vi "DrawInvaders_Intensity.vi"(4 "Step_V":i32, 6 "Step_H":i32, 7 "Clear":bool, 9 "InitCluster_IN":T1, 11 "InvaderArray":bool[][](array[boolean])=[[TRUE, TRUE, TRUE, TRUE, TRUE, TRUE, TRUE, TRUE, TRUE, TRUE], [TRUE, TRUE, TRUE, TRUE, TRUE, TRUE, TRUE, TRUE, TRUE, TRUE], [TRUE, TRUE, TRUE, TRUE, TRUE, TRUE, TRUE, TRUE, TRUE, TRUE], [TRUE, TRUE, TRUE, TRUE, TRUE, TRUE, TRUE, TRUE, TRUE, TRUE], [TRUE, TRUE, TRUE, TRUE, TRUE, TRUE, TRUE, TRUE, TRUE, TRUE]]) -> (1 "InitCluster_OUT":T1, 3 "InvaderPosArray":T9(array[cluster]))   [LabVIEW 2022 SP3]
uses:
  InitCluster.ctl
  CharacterCluster.ctl
  <vilib>/picture/picture.llb/imagedata.ctl
  ShotInitCluster.ctl
  <vilib>/Utility/miscctls.llb/LVPositionTypeDef.ctl
  <vilib>/Utility/miscctls.llb/LVBoundsTypeDef.ctl
  ShotCluster.ctl
  move_dir_ud.ctl
panel:
  out "IG":u8[][](graph)
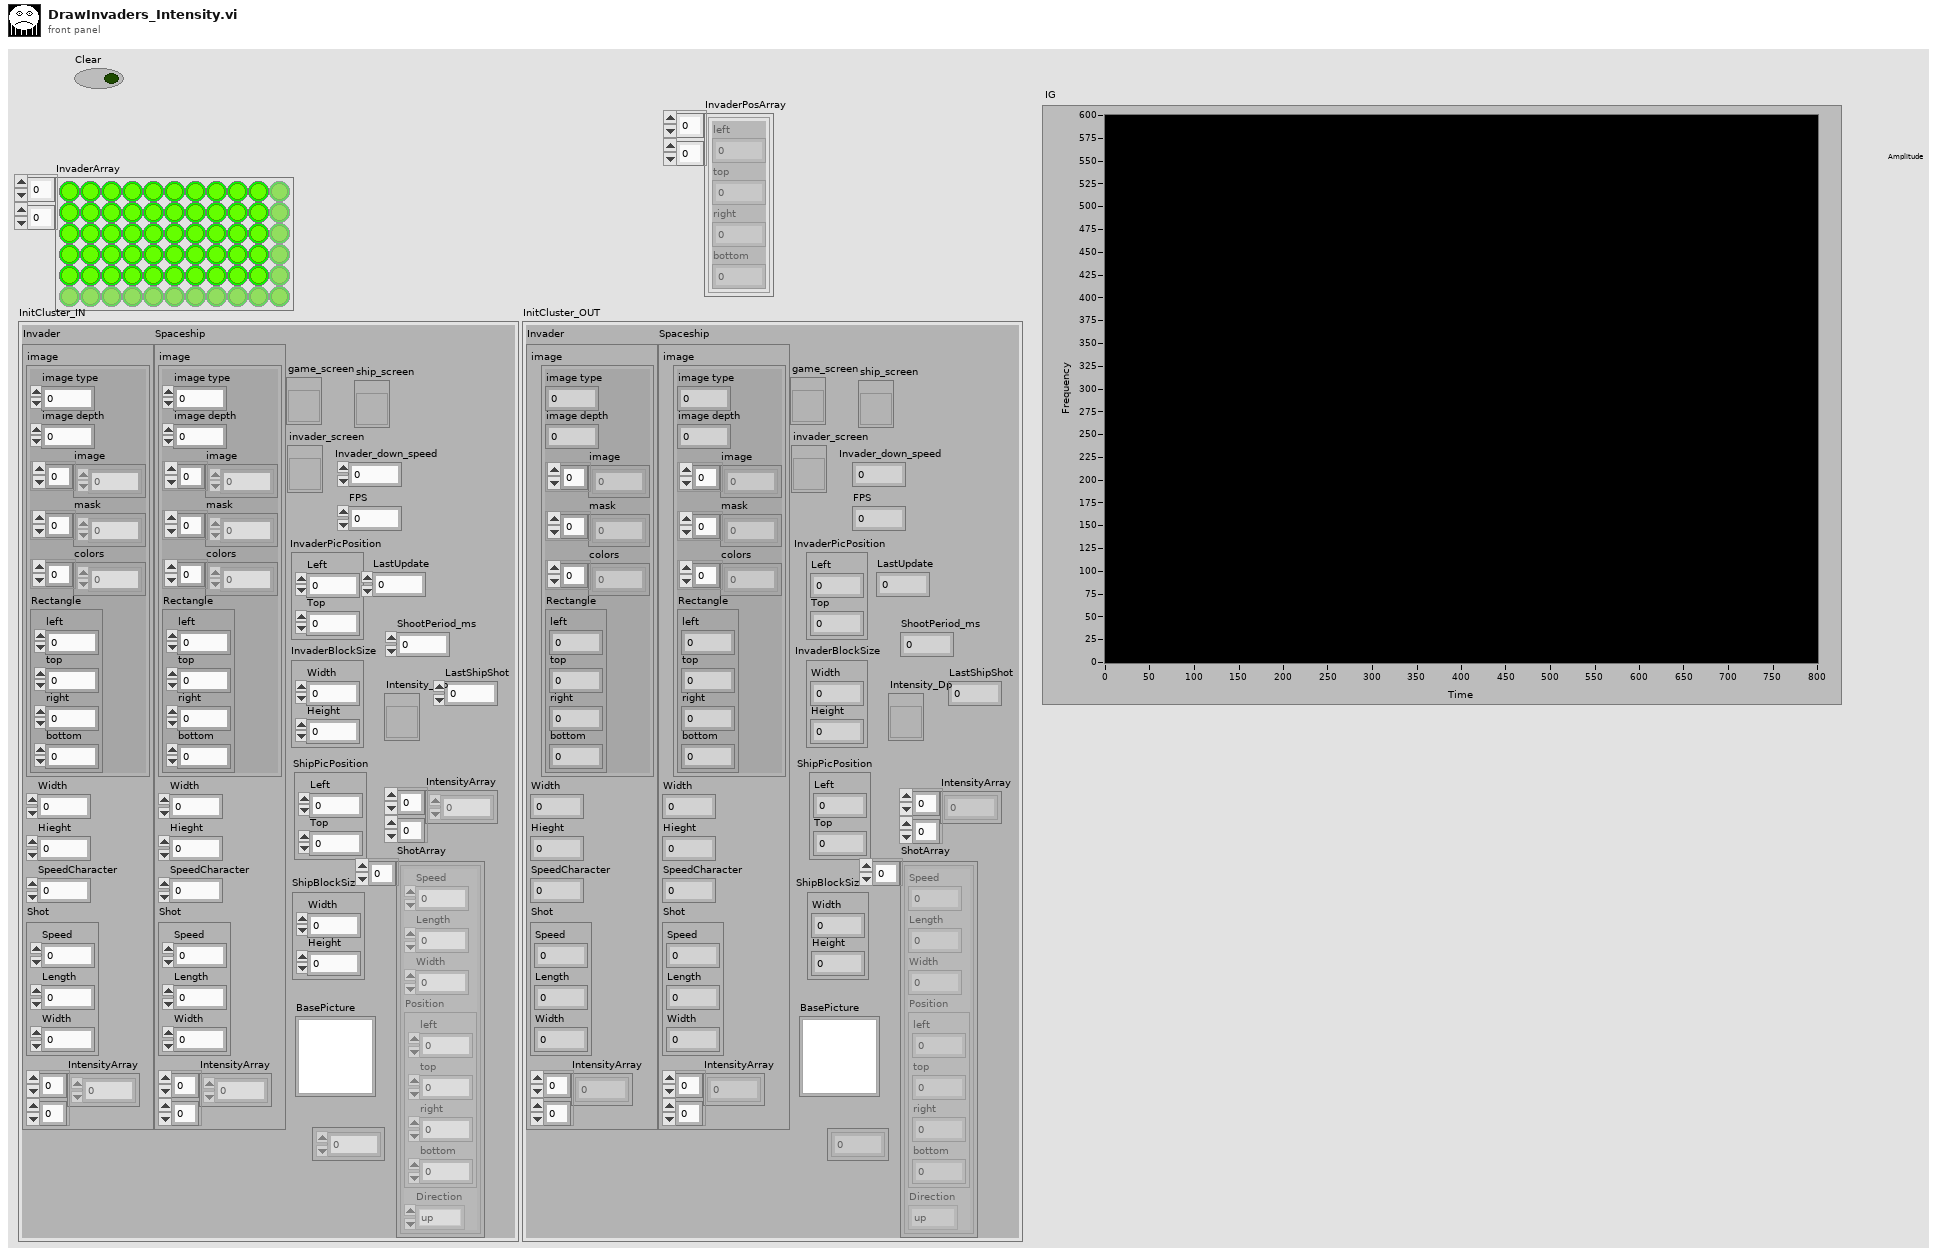
[diagram p1: front panel]
types:
  T1 = typedef "InitCluster.ctl" = cluster{"Invader":T2, "Spaceship":T2, "game_screen":refnum<vi>, "BasePicture":picture, "invader_screen":refnum<vi>, "InvaderPicPosition":T5, "Invader_down_speed":i16, "FPS":u16, "InvaderBlockSize":T6, "ship_screen":refnum<vi>, "ShipBlockSize":T6, "ShipPicPosition":T5, "LastUpdate":u32, "Intensity_Dp":refnum<vi>, "IntensityArray":u8[][], "ShotArray":T7[], "InvaderShotTimeArray":u32[], "ShootPeriod_ms":i32, "LastShipShot":u32}
  T2 = typedef "CharacterCluster.ctl" = cluster{"image":T3, "Width":u32, "Hieght":u32, "SpeedCharacter":u32, "Shot":T4, "IntensityArray":u8[][]}
  T3 = typedef "imagedata.ctl" = cluster{"image type":i32, "image depth":i32, "image":u8[], "mask":u8[], "colors":u32[], "Rectangle":cluster{"left":i16, "top":i16, "right":i16, "bottom":i16}}
  T4 = typedef "ShotInitCluster.ctl" = cluster{"Speed":u32, "Length":u32, "Width":u32}
  T5 = typedef "LVPositionTypeDef.ctl" = cluster{"Left":i32, "Top":i32}
  T6 = typedef "LVBoundsTypeDef.ctl" = cluster{"Width":u32, "Height":u32}
  T7 = typedef "ShotCluster.ctl" = cluster{"Speed":u32, "Length":u32, "Width":u32, "Position":cluster{"left":i16, "top":i16, "right":i16, "bottom":i16}, "Direction":T8}
  T8 = typedef "move_dir_ud.ctl" = enum16{"up", "down"}
  T9 = cluster{"left":i16, "top":i16, "right":i16, "bottom":i16}[][]
  T10 = cluster{"left":i16, "top":i16, "right":i16, "bottom":i16}
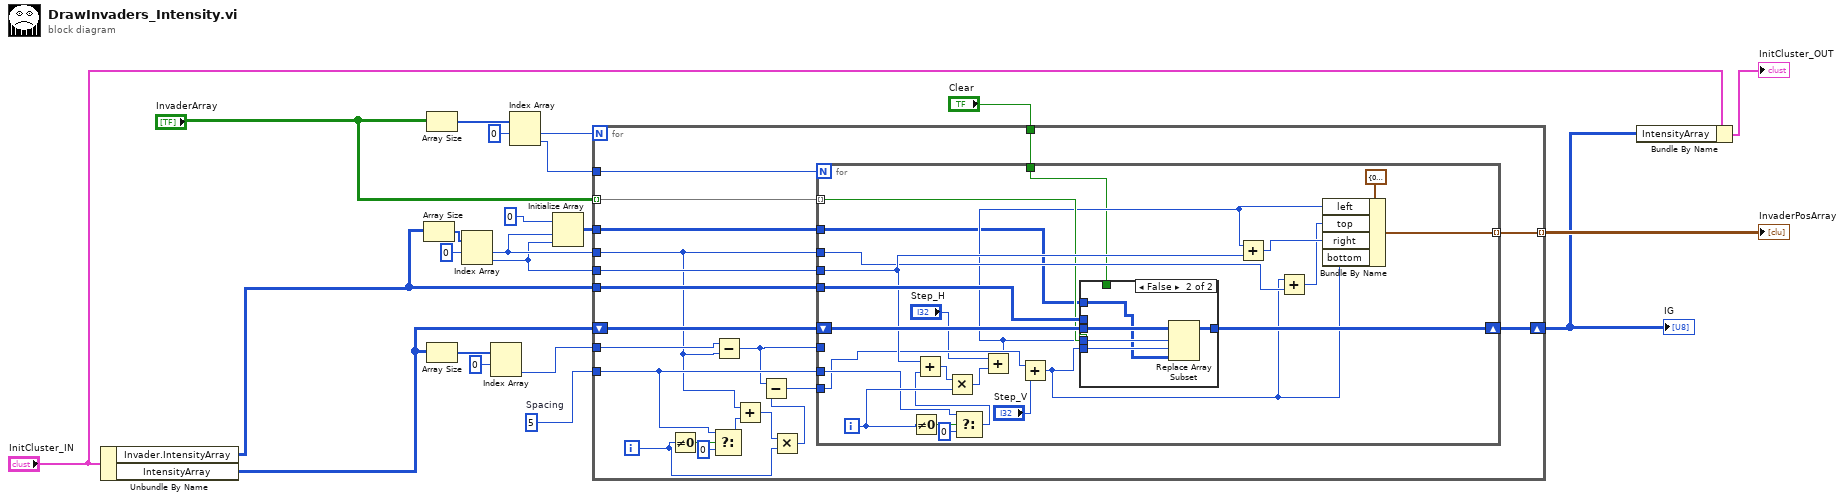
[diagram p0: block diagram]
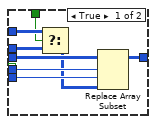
[diagram p2: hidden frame]
diagram:
  w22 = u8 5  # Spacing
  n1 = Unbundle By Name("InitCluster_IN") -> ("Invader.IntensityArray"=w12:u8[][], "IntensityArray"=w4:u8[][])
  n2 = Array Size(array=w12) -> (size(s)=w20:i32[])
  n3 = Array Size(array="InvaderArray") -> (size(s)=w18:i32[])
  n4 = Array Size(array=w4) -> (size(s)=w6:i32[])
  n5 = Index Array(array=w20, index #1=0 ("index")) -> (element #1=w11:i32, element #2=w10:i32)  [unwired: 1 in]
  n6 = Index Array(array=w6, index #1=0 ("index")) -> (element #2=w13:i32)  [unwired: 1 in, 1 out]
  n7 = Index Array(array=w18, index #1=0 ("index")) -> (element #1=w16:i32, element #2=w15:i32)  [unwired: 1 in]
  n8 = Initialize Array(u8 0, w11, w10) -> (w8:u8[][])
  n9 = for {
    N: w16 -> [_]
    tunnel: w12 -> [w42]
    shift-right: [w40] -> w1
    shift-left: w4 -> [w41]
    tunnel: w22 -> [w35]
    tunnel: w11 -> [w28]
    tunnel: w10 -> [w39]
    tunnel: w13 -> [w30]
    tunnel: [w27] -> w19 mode=indexing
    tunnel: w15 -> [w26]
    tunnel: "InvaderArray" -> [w25] mode=indexing
    tunnel: w8 -> [w24]
    tunnel: "Clear" -> [w23]
    i -> [w32]
    n10 = Not Equal To 0?(x=w32) -> (x != 0?=w37:bool)
    n11 = Select(t=w35, s=w37, f=u8 0) -> (s? t:f=w36:u8)
    n12 = Subtract(x=w30, y=w28) -> (x-y=w29:i32)
    n13 = Add(x=w28, y=w36) -> (x+y=w33:i32)
    n14 = Multiply(x=w33, y=w32) -> (x*y=w31:i32)
    n15 = Subtract(x=w29, y=w31) -> (x-y=w34:i32)
    n16 = for {
      N: w26 -> [_]
      tunnel: w42 -> [w64]
      tunnel: w35 -> [w60]
      shift-right: [w65] -> w40
      shift-left: w41 -> [w66]
      tunnel: w28 -> [w54]
      tunnel: w39 -> [w56]
      tunnel: w29 -> [_]
      tunnel: w34 -> [w50]
      tunnel: [w53] -> w27 mode=indexing
      tunnel: w25 -> [w51] mode=indexing
      tunnel: w24 -> [w44]
      tunnel: w23 -> [w43]
      i -> [w62]
      n17 = Not Equal To 0?(x=w62) -> (x != 0?=w61:bool)
      n18 = Select(t=w60, s=w61, f=u8 0) -> (s? t:f=w58:u8)
      n19 = Add(x=w56, y=w58) -> (x+y=w63:i32)
      n20 = Multiply(x=w63, y=w62) -> (x*y=w47:i32)
      n21 = Add(x="Step_H", y=w47) -> (x+y=w45:i32)
      n22 = Add(x=w50, y="Step_V") -> (x+y=w48:i32)
      n23 = case shown="False" w51 {
        tunnel: w66 -> [w74 w79]
        tunnel: [w73 w78] -> w65
        tunnel: w64 -> [w69 _]
        tunnel: w45 -> [w72 w77]
        tunnel: w48 -> [w71 w76]
        tunnel: w44 -> [w70 w75]
        tunnel: w43 -> [w68 _]
        frame True {
          n24 = Select(t=w70, s=w68, f=w69) -> (s? t:f=w67:u8[][])
          n25 = Replace Array Subset(array=w74, new element=w67, index (row)=w72, index (col)=w71) -> (w73:u8[][])
        }
        frame False {
          n26 = Replace Array Subset(array=w79, new element=w75, index (row)=w77, index (col)=w76) -> (w78:u8[][])
        }
      }
      n27 = Add(x=w45, y=w56) -> (x+y=w55:i32)
      n28 = Add(x=w48, y=w54) -> (x+y=w52:i32)
      n29 = Bundle By Name(cluster=T10 {"left"=0, "top"=0, "right"=0, "bottom"=0} ("Rectangle"), "left"=w45, "top"=w52, "right"=w55, "bottom"=w48) -> (w53:T10)
    }
  }
  "InvaderPosArray" <- w19
  "IG" <- w1
  n30 = Bundle By Name(cluster="InitCluster_IN", "IntensityArray"=w1) -> (→"InitCluster_OUT":T1)
